vi "GetServiceRequestEnableRegister.vi"(8 "Error In":errorcluster, 11 "Keithley 2602 In":refnum<visa-resource-name>) -> (0 "Error Out":errorcluster, 2 "Service Request Enable Register":bool[](array[boolean]), 3 "Keithley 2602 Out":refnum<visa-resource-name>)   [LabVIEW 2012, in "Keithley-2602.lvlib"]
uses:
  Keithley-2602.lvlib
panel:
  # "MSB"
  # "EAV"
  # "MAV"
  # "RQS"
  # "SSB"
  # "QSB"
  # "ESB"
  # "OSB"
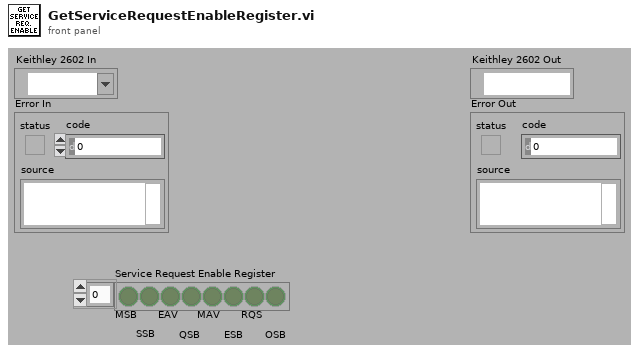
[diagram p1: front panel]
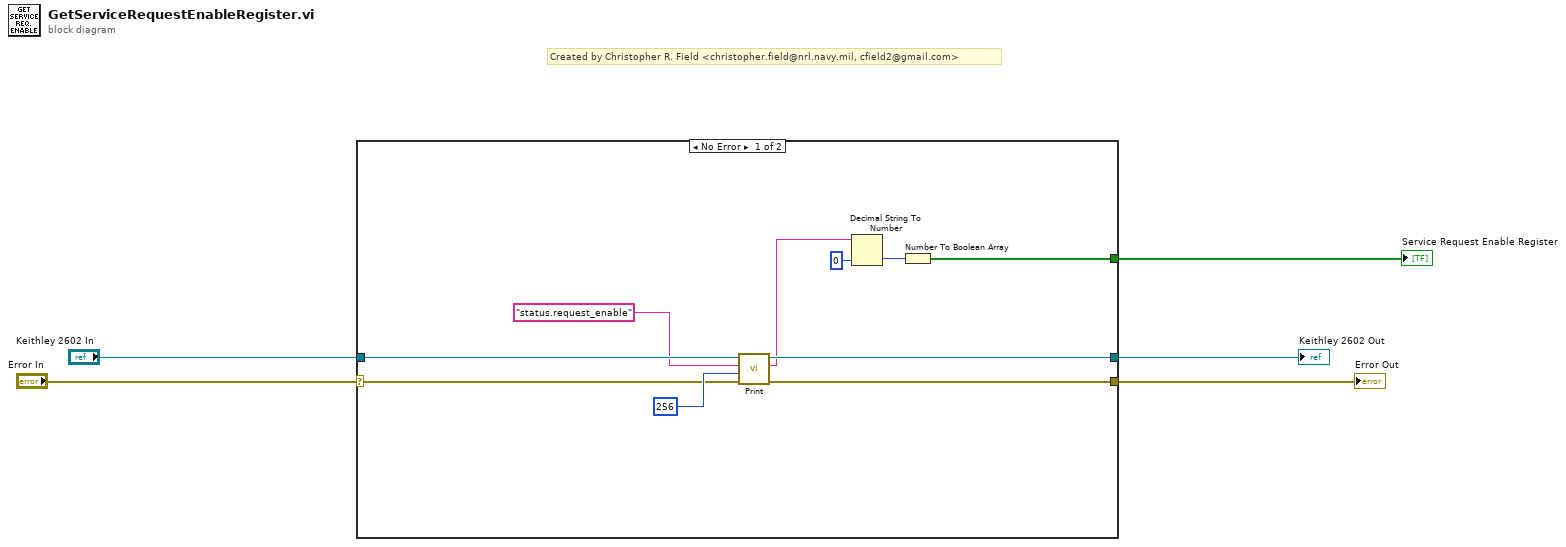
[diagram p0: block diagram]
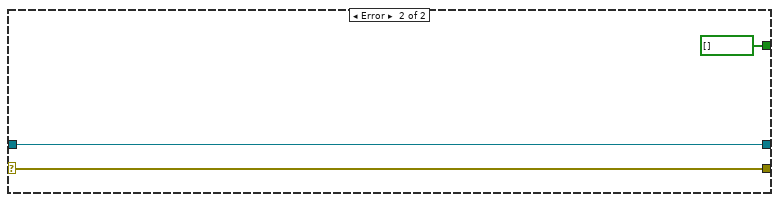
[diagram p2: hidden frame]
diagram:
  # "Created by Christopher R. Field <christopher.field@nrl.navy.mil, cfield2@gmail.com>"
  n1 = case shown="No Error" "Error In" {
    selector: "Error In" -> [w6 w17]
    tunnel: "Keithley 2602 In" -> [w15 w18]
    tunnel: [w12 w18] -> w4
    tunnel: [w11 w17] -> w3
    tunnel: [w7 bool[] [] ("Boolean array")] -> w2
    frame No Error {
      n2 = call "Print.vi"("Error In"=w6, "Byte Count"=u32 256, "Attribute"="status.request_enable" ("write buffer"), "Kiethley 2602 In"=w15) -> ("Error Out"=w11:errorcluster, "Output"=w10:string, "Keithley 2602 Out"=w12:refnum<visa-resource-name>)  [unwired: 5 in]
      n3 = Decimal String To Number(string=w10, default (0L)=u16 0 ("default (0 I32)")) -> (number=w8:u16)  [unwired: 1 in, 1 out]
      n4 = Number To Boolean Array(number=w8) -> (Boolean array=w7:bool[])
    }
    frame Error {
    }
  }
  "Keithley 2602 Out" <- w4
  "Error Out" <- w3
  "Service Request Enable Register" <- w2
